vi "Get1DSortMap.vi"(1 "Sorted":dbl[](array[numeric]), 2 "Original":dbl[](array[numeric])) -> (0 "SortMap":cluster{i32, "index of element":i32}[](array[cluster]))   [LabVIEW 2010]
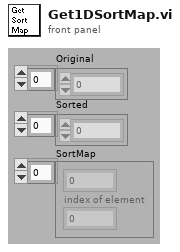
[diagram p1: front panel]
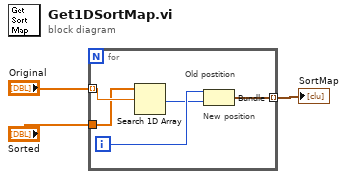
[diagram p0: block diagram]
diagram:
  n1 = for {
    tunnel: "Original" -> [w8] mode=indexing
    tunnel: "Sorted" -> [w7]
    tunnel: [w4] -> w1 mode=indexing
    i -> [w6]
    # "New position"
    # "Old postition"
    n2 = Search 1D Array(1D array=w7, element=w8) -> (index of element=w5:i32)  [unwired: 1 in]
    n3 = Bundle(w6, "index of element"=w5) -> (w4:cluster{i32, "index of element":i32})  [unwired: 1 in]
  }
  "SortMap" <- w1
